vi "Valve test.vi"() -> ()   [LabVIEW 2016]
uses:
  <vilib>/DAQmx/write.llb/DAQmx Write (Digital 1D Bool 1Chan 1Samp).vi
  <vilib>/DAQmx/read.llb/DAQmx Read (Analog 1D DBL NChan 1Samp).vi
  <vilib>/DAQmx/create/channels.llb/DAQmx Create Channel (AI-Current-Basic).vi
  <vilib>/DAQmx/create/channels.llb/DAQmx Create Channel (DO-Digital Output).vi
  <vilib>/DAQmx/miscellaneous.llb/DAQmx Fill In Error Info.vi
  <resource>/objmgr/daqmx.rc
panel:
  in  "Vacuum":bool
  in  "Tube Open":bool
  in  "Stop Button":bool
  out "Tube Pressure":dbl[][](graph)
  in  "Purge":bool
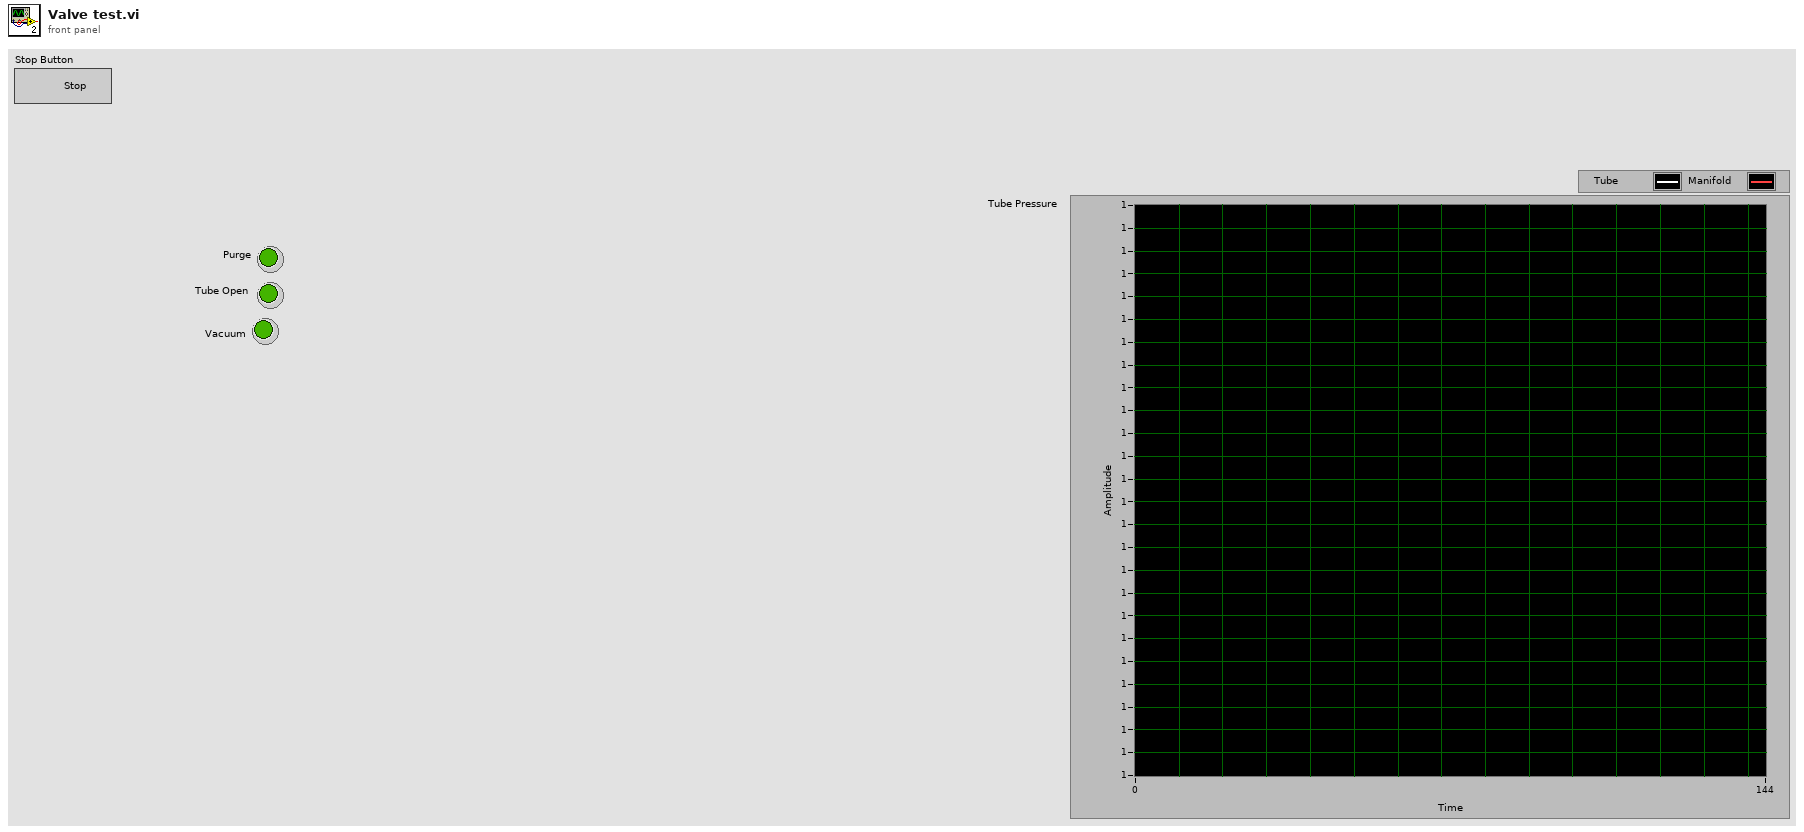
[diagram p1: front panel]
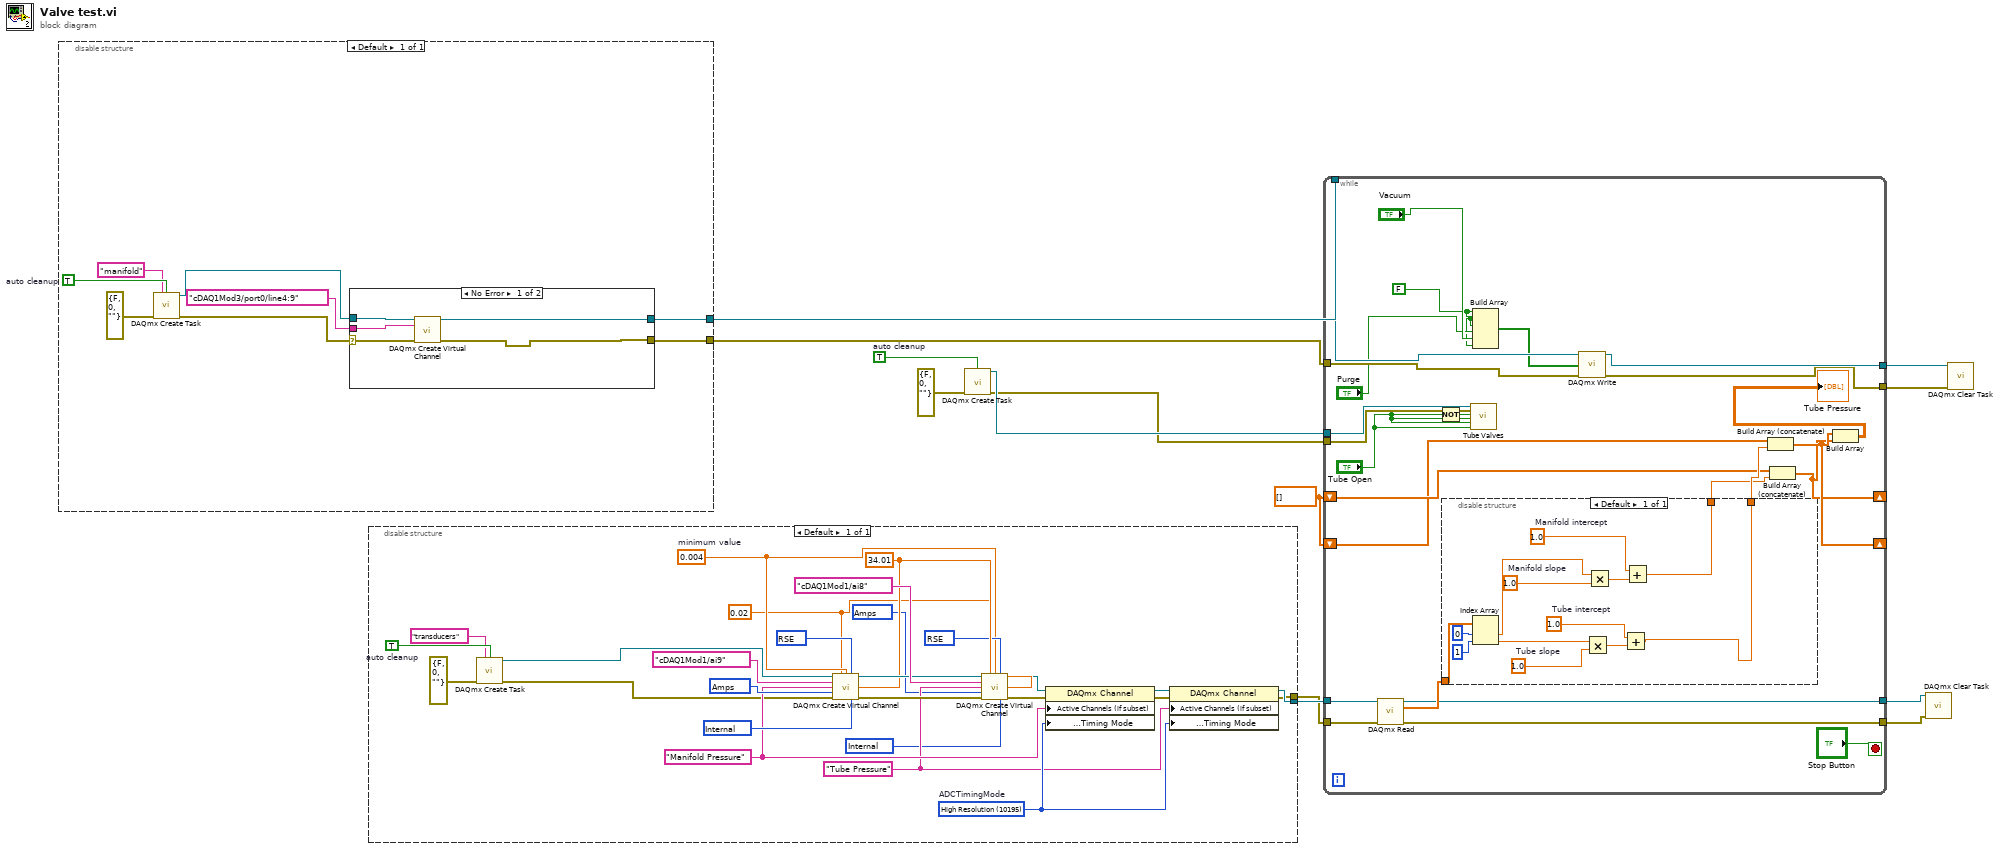
[diagram p0: block diagram]
diagram:
  w5 = dbl[] []
  w12 = TRUE  # auto cleanup
  n1 = disable-structure shown="Default" {
    disable-tunnel: [w15] -> w4
    disable-tunnel: [w14] -> w3
    frame Enabled {
      w21 = TRUE  # auto cleanup
      n2 = call <vilib>:"DAQmx Create Task.vi"("new task name"="manifold", "auto cleanup"=w21, "error in"=errorcluster {"status"=FALSE, "code"=0, "source"=""}) -> ("task out"=w17:refnum<k21>, "error out"=w16:errorcluster)  [unwired: 11 in]
      n3 = case shown="No Error" w16 {
        selector: w16 -> [w25 w28]
        tunnel: [w22 w28] -> w15
        tunnel: tag "cDAQ1Mod3/port0/line4:9" ("lines") -> [w26 _]
        tunnel: w17 -> [w24 w27]
        tunnel: [w23 w27] -> w14
        frame No Error {
          n4 = call-poly <vilib>:"DAQmx Create Virtual Channel.vi"("task in"=w24, "lines"=w26, "error in"=w25) -> ("task out"=w23:refnum<k21>, "error out"=w22:errorcluster)  [unwired: 11 in]
        }
        frame Error {
        }
      }
    }
  }
  n5 = disable-structure shown="Default" {
    disable-tunnel: [w30] -> w9
    disable-tunnel: [w29] -> w8
    frame Enabled {
      w35 = 10200 items=["default"=-1, "Internal"=10200, "External"=10167] ("shunt resistor location")
      w36 = 10342 items=["Amps"=10342, "From Custom Scale"=10065] ("units")
      w37 = 10083 items=["default"=-1, "RSE"=10083, "NRSE"=10078, "Differential"=10106, "Pseudodifferential"=12529] ("input terminal configuration")
      w41 = 10195 items=["High Resolution"=10195, "High Speed"=14712, "Best 50 Hz Rejection"=14713, "Best 60 Hz Rejection"=14714]  # ADCTimingMode
      w40 = "Tube Pressure" ("name to assign")
      w42 = "Manifold Pressure" ("name to assign")
      w46 = 34.01 ("external shunt resistor value")
      w45 = 10200 items=["default"=-1, "Internal"=10200, "External"=10167] ("shunt resistor location")
      w51 = 10083 items=["default"=-1, "RSE"=10083, "NRSE"=10078, "Differential"=10106, "Pseudodifferential"=12529] ("input terminal configuration")
      w34 = 0.004  # minimum value
      w33 = 0.02 ("maximum value")
      w49 = 10342 items=["Amps"=10342, "From Custom Scale"=10065] ("units")
      w54 = TRUE  # auto cleanup
      n6 = call <vilib>:"DAQmx Create Task.vi"("new task name"="transducers", "auto cleanup"=w54, "error in"=errorcluster {"status"=FALSE, "code"=0, "source"=""}) -> ("task out"=w32:refnum<k21>, "error out"=w31:errorcluster)  [unwired: 11 in]
      n7 = call-poly <vilib>:"DAQmx Create Virtual Channel.vi"("task in"=w32, "maximum value"=w33, "minimum value"=w34, "input terminal configuration"=w51, "physical channels"=tag "cDAQ1Mod1/ai9", "name to assign"=w42, "external shunt resistor value"=w46, "units"=w49, "error in"=w31, "shunt resistor location"=w45) -> ("task out"=w47:refnum<k21>, "error out"=w48:errorcluster)  [unwired: 4 in]
      n8 = call-poly <vilib>:"DAQmx Create Virtual Channel.vi"("task in"=w47, "maximum value"=w33, "minimum value"=w34, "input terminal configuration"=w37, "physical channels"=tag "cDAQ1Mod1/ai8", "name to assign"=w40, "external shunt resistor value"=w46, "units"=w36, "error in"=w48, "shunt resistor location"=w35) -> ("task out"=w39:refnum<k21>, "error out"=w38:errorcluster)  [unwired: 4 in]
      n9 = property class="DAQmx Channel"(reference=w39, error in=w38, "Active Channels (if subset)"=w42, "Analog Input:General Properties:Digitizer/ADC:Timing Mode"=w41) -> (reference out=w43:refnum<k21>, error out=w44:errorcluster)
      n10 = property class="DAQmx Channel"(reference=w43, error in=w44, "Active Channels (if subset)"=w40, "Analog Input:General Properties:Digitizer/ADC:Timing Mode"=w41) -> (reference out=w30:refnum<k21>, error out=w29:errorcluster)
    }
  }
  n11 = call <vilib>:"DAQmx Create Task.vi"("auto cleanup"=w12, "error in"=errorcluster {"status"=FALSE, "code"=0, "source"=""}) -> ("task out"=w11:refnum<k21>, "error out"=w10:errorcluster)  [unwired: 12 in]
  n12 = while {
    tunnel: w11 -> [w79]
    tunnel: w10 -> [w78]
    shift-right: [w69] -> _
    shift-left: w5 -> [w67]
    tunnel: w9 -> [w75]
    tunnel: w8 -> [w74]
    tunnel: [w73] -> w7
    tunnel: [w72] -> w6
    shift-right: [w70] -> _
    shift-left: w5 -> [w65]
    tunnel: w4 -> [w62]
    tunnel: w3 -> [w63]
    tunnel: [w57] -> w2
    tunnel: [w56] -> w1
    stop <- "Stop Button" stop-if-true
    w58 = FALSE ("element")
    n13 = call-poly <vilib>:"DAQmx Read.vi"("task/channels in"=w75, "error in"=w74) -> ("task out"=w72:refnum<k21>, "data"=w76:dbl[], "error out"=w73:errorcluster)  [unwired: 11 in]
    n14 = Not(x="Tube Open") -> (.not. x?=w66:bool)
    n15 = disable-structure shown="Default" {
      disable-tunnel: w76 -> [w91]
      disable-tunnel: [w81] -> w71
      disable-tunnel: [w82] -> w68
      frame Enabled {
        w86 = 1.0  # Tube intercept
        w85 = 1.0  # Tube slope
        w90 = 1.0  # Manifold intercept
        w88 = 1.0  # Manifold slope
        n16 = Index Array(array=w91, index #1=0 ("index"), index #2=1 ("index")) -> (element #1=w83:dbl, element #2=w84:dbl)
        n17 = Multiply(x=w84, y=w85) -> (x*y=w87:dbl)
        n18 = Multiply(x=w83, y=w88) -> (x*y=w89:dbl)
        n19 = Add(x=w86, y=w87) -> (x+y=w81:dbl)
        n20 = Add(x=w90, y=w89) -> (x+y=w82:dbl)
      }
    }
    n21 = call "Tube Valves.vi"("task in"=w79, "Error In"=w78, "Tube Inlet"=w66, "Mix Inlet"="Tube Open", "Mix Outlet"="Tube Open", "Tube Outlet"="Tube Open") -> ()  [unwired: 9 in, 5 out]
    n22 = Build Array(w58, w58, w58, "Purge", "Vacuum", w58) -> (w61:bool[])
    n23 = call-poly <vilib>:"DAQmx Write.vi"("task/channels in"=w63, "data"=w61, "error in"=w62) -> ("task out"=w57:refnum<k21>, "error out"=w56:errorcluster)  [unwired: 10 in, 1 out]
    n24 = Build Array (concatenate)(w65, w71) -> (w70:dbl[])
    n25 = Build Array (concatenate)(w67, w68) -> (w69:dbl[])
    n26 = Build Array(w70, w69) -> (→"Tube Pressure":dbl[][])
  }
  n27 = call <vilib>:"DAQmx Clear Task.vi"("task in"=w6, "error in"=w7) -> ()  [unwired: 13 in, 1 out]
  n28 = call <vilib>:"DAQmx Clear Task.vi"("task in"=w2, "error in"=w1) -> ()  [unwired: 13 in, 1 out]
